vi "A1 处理函数CCD2.vi"(8 "error in (no error)":errorcluster caption="错误输入（无错误）", 10 "Image Name":string="I1", 11 "ParamsUI":T2 caption="参数界面" {"Exposure Values" scale=0.0..200000.0}) -> (0 "error out":errorcluster caption="错误输出", 1 "Session out":T1, 2 "Buffer Number Out":u32, 3 "Image out":T3(plugin-control))   [LabVIEW 2017]
uses:
  <resource>/objmgr/imaqdx.rc
  <vilib>/vision/driver/NI_Vision_Acquisition_Software.lvlib
  <vilib>/userdefined/High Color/IMAQdx.ctl
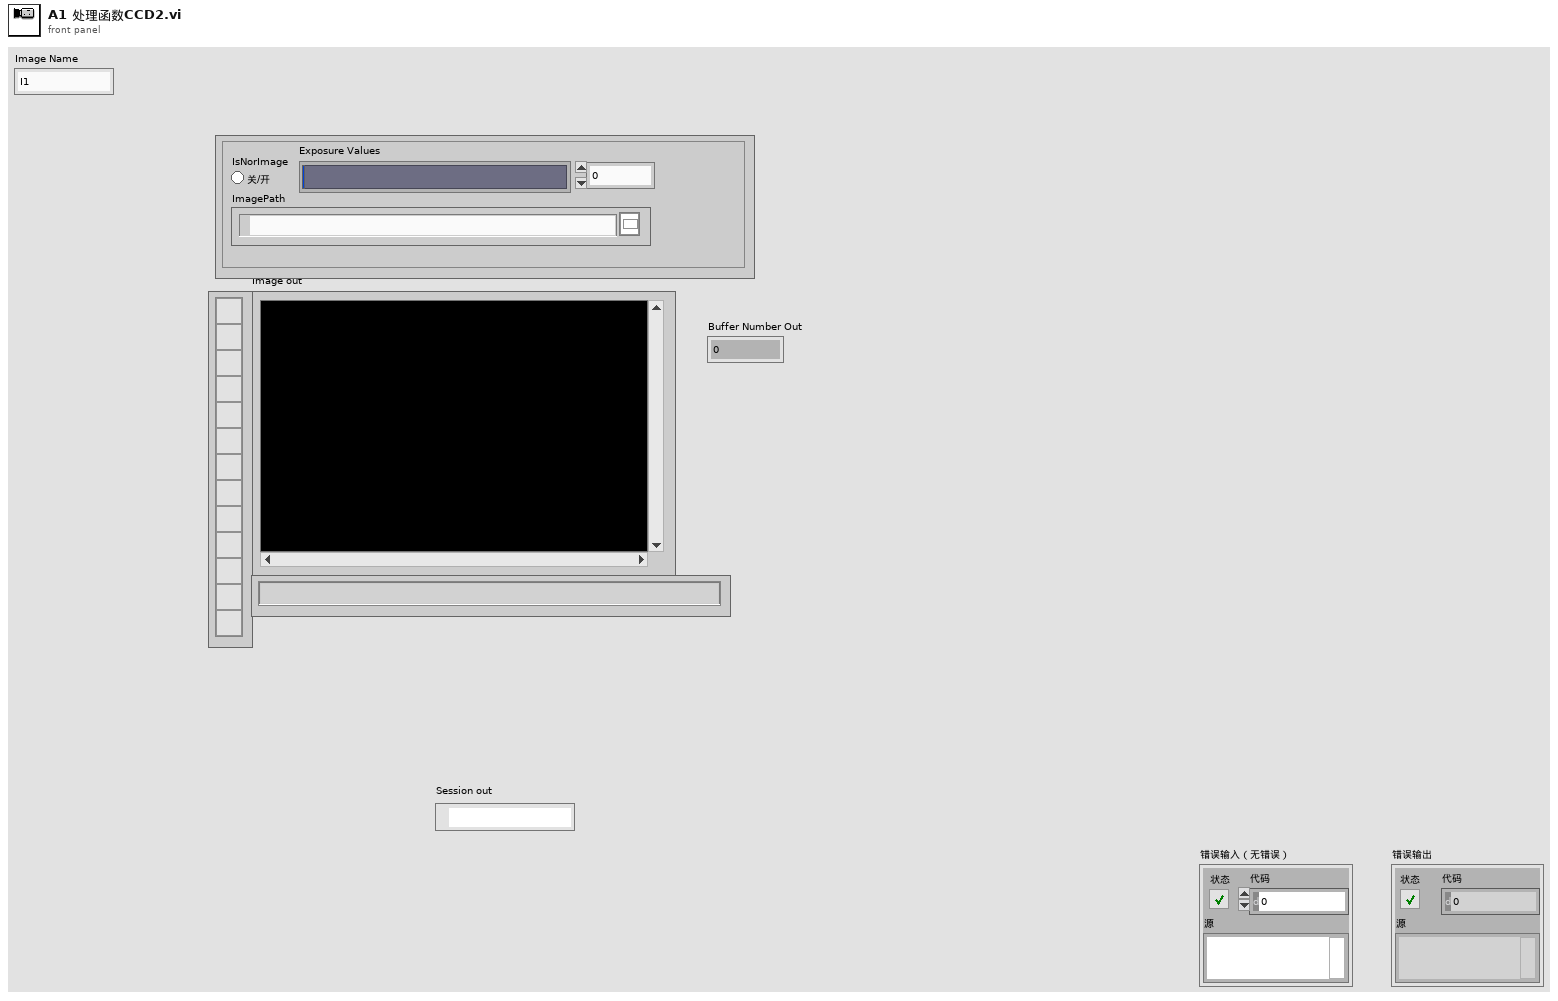
[diagram p1: front panel]
types:
  T1 = typedef "IMAQdx.ctl" = refnum<k21>
  T2 = cluster{"IsNorImage":bool, "Exposure Values":u32, "ImagePath":path}
  T3 = typedef "IMAQ Image.ctl" = refnum<image>
  T4 = typedef "Image Type" = u32
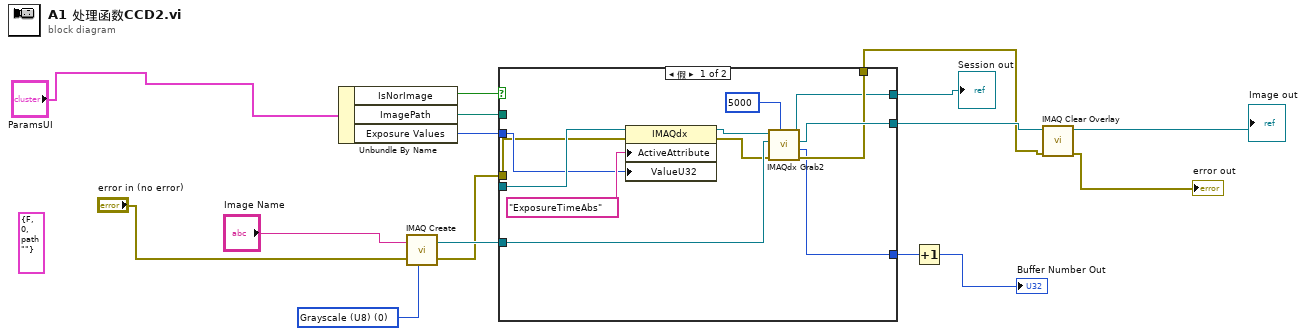
[diagram p0: block diagram]
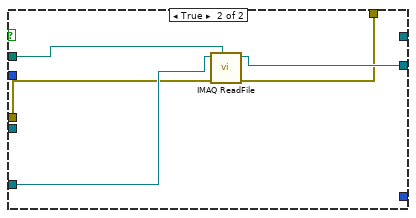
[diagram p2: hidden frame]
diagram:
  w11 = T4 0 items=["Grayscale (U8)", "Grayscale (I16)", "Grayscale (SGL)", "Complex (CSG)", "RGB (U32)", "HSL (U32)", "RGB (U64)", "Grayscale (U16)"] ("Image Type")
  (unwired) T2 {"IsNorImage"=FALSE, "Exposure Values"=0, "ImagePath"=path ""} ("ParamsUI")
  n1 = Unbundle By Name("ParamsUI") -> ("IsNorImage"=w17:bool, "ImagePath"=w16:path, "Exposure Values"=w15:u32)
  n2 = call "IMAQ Create"("Image Name"="Image Name", "Image Type"=w11, "error in (no error)"="error in (no error)") -> ("New Image"=w13:T3, "error out"=w2:errorcluster)  [unwired: 2 in]
  n3 = case shown="假" w17 {
    tunnel: w16 -> [_ w34]
    tunnel: [w23 w33] -> w10
    tunnel: w15 -> [w27 _]
    tunnel: [w29 _] -> w1
    tunnel: w13 -> [w25 w32]
    tunnel: w2 -> [w22 w31]
    tunnel: [w21 w30] -> w9
    tunnel: [w20 _] -> w6
    tunnel: [w19 _] -> w4
    frame False {
      n4 = property class="IMAQdx"(reference=w29, error in=w22, "ActiveAttribute"="ExposureTimeAbs", "ValueU32"=w27) -> (reference out=w26:T1, error out=w24:errorcluster)
      n5 = call <vilib>:"IMAQdx Grab2.vi"("Timeout (ms)"=5000, "error in"=w24, "Image In"=w25, "Session In"=w26) -> ("error out"=w21:errorcluster, "Buffer Number Out"=w20:u32, "Image Out"=w23:T3, "Session Out"=w19:T1)  [unwired: 4 in]
    }
    frame True {
      n6 = call "IMAQ ReadFile"("File Path"=w34, "error in (no error)"=w31, "Image"=w32) -> ("error out"=w30:errorcluster, "Image Out"=w33:T3)  [unwired: 4 in, 3 out]
    }
  }
  "Session out" <- w4
  n7 = Increment(x=w6) -> (x+1=→"Buffer Number Out":u32)
  n8 = call "IMAQ Clear Overlay"("error in (no error)"=w9, "Image"=w10) -> ("error out"=→"error out":errorcluster, "Image Out"=→"Image out":T3)  [unwired: 8 in]
